vi "UpdateAOUIcontrol.vi"(8 "error in (no error)":errorcluster, 9 "String":string, 10 "Numeric":dbl, 11 "Data Value Reference in":T1) -> (0 "error out":errorcluster, 3 "Data Value Reference out":T1)   [LabVIEW 2022 SP3, in "TopLevel.lvclass"]
uses:
  TopLevel.lvclass
  <vilib>/TELLC/Dynamic CVT API/TD Dynamic CVT DVR--ref.ctl
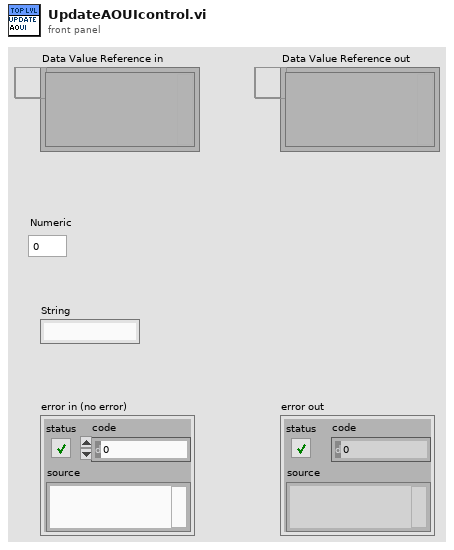
[diagram p1: front panel]
types:
  T1 = typedef "TD Dynamic CVT DVR--ref.ctl" = refnum<data-value>
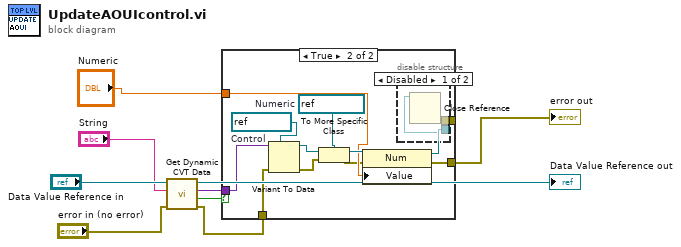
[diagram p0: block diagram]
diagram:
  n1 = call <vilib>:"Get Dynamic CVT Data.vi"("error in (no error)"="error in (no error)", "DataName"="String", "dCVT DVR"="Data Value Reference in") -> ("error out"=w7:errorcluster, "found"=w5:bool, "value"=w6:variant, "dCVT DVR out"=→"Data Value Reference out":T1)  [unwired: 5 in]
  n2 = case shown="True" w5 {
    tunnel: w6 -> [_ w22]
    tunnel: w7 -> [w10 w17]
    tunnel: "Numeric" -> [_ w15]
    tunnel: [w10 w12] -> w8
    tunnel: [_ w11] -> _
    frame False {
    }
    frame True {
      w20 = refnum<vi> refnum  # Numeric
      w21 = refnum<vi> refnum  # Control
      n3 = Variant To Data(error in=w17, type=w21, Variant=w22) -> (data=w19:refnum<vi>, error out=w18:errorcluster)
      n4 = To More Specific Class(target class=w20, reference=w19, error in=w18) -> (specific class reference=w16:refnum<vi>, error out=w14:errorcluster)
      n5 = property class="Num"(reference=w16, error in=w14, "Value"=w15) -> (reference out=w13:refnum<vi>, error out=w12:errorcluster)
      n6 = disable-structure shown="Disabled" {
        disable-tunnel: w13 -> [w24 _]
        disable-tunnel: [w23 _] -> w11
        frame Disabled {
          n7 = Close Reference(reference=w24) -> (error out=w23:errorcluster)  [unwired: 1 in]
        }
        frame Enabled {
        }
      }
    }
  }
  "error out" <- w8
